vi "Autonomous Independent.vi"   [LabVIEW 2017]
doc: "This VI is called when autonomous begins, and will automatically be terminated when autonomous ends. You can carry out timed or sensor driven robot movement independently without needing to return to the caller."
uses:
  <vilib>/Rock Robotics/WPI/SafetyOutput/WPI_SafetyOutputConfigMenu.ctl
  <vilib>/Rock Robotics/WPI/ThirdParty/Phoenix-LabVIEW/Motor Controller/Controls/CTRE_Phoenix_MotorControl_ControlMode.ctl
  <vilib>/Rock Robotics/WPI/Utilities/WPI_GetSetVariantRefNum.vi
  Robot Global Data.vi
  <vilib>/Rock Robotics/WPI/RobotDrive/WPI_RobotDriveArcadeDrive_Standard(NoSaturation).vi
  <vilib>/Rock Robotics/WPI/RobotDrive/WPI_RobotDriveMecanumDrive_Cartesian.vi
  <vilib>/Rock Robotics/WPI/RobotDrive/WPI_RobotDriveMecanumDrive_Polar.vi
panel:
  # "Be sure to right-click and choose Data Operations>>Make Current Value default if you want to save the array values with the VI"
types:
  T1 = typedef "WPI_SafetyOutputConfigMenu.ctl" = enum16{"Enable", "Disable"}
  T2 = typedef "WPI_RobotDriveDevRef.ctl" = cluster{"DevStatus":errorcluster, "Motors[]":T3[], "Square Inputs":bool, "Max Output":dbl}
  T3 = typedef "WPI_MotorControlDeviceRef.ctl" = cluster{"DeviceStatus":errorcluster, "Type":T4, "PWM":cluster{"PWM Channel":T5, "DeadBand":T6}, "CAN":cluster{"Device Number":u8, "SetOutput VI Ref":variant, "GetOutput VI Ref":variant, "Enable VI Ref":variant, "Disable VI Ref":variant, "Data":variant}, "Invert":bool, "DIO PWM":cluster{"PWM \"Enable\" Channel":T5, "DIOChannel":T7, "PWM Rate":dbl}}
  T4 = typedef "WPI_MotorControlType.ctl" = enum16{"PWM", "CAN", "DIO PWM"}
  T5 = typedef "FPGA_DIOPWMChannel.ctl" = enum8{"PWM 0", "PWM 1", "PWM 2", "PWM 3", "PWM 4", "PWM 5", "PWM 6", "PWM 7", "PWM 8", "PWM 9", "PWM MXP 0", "PWM MXP 1", "PWM MXP 2", "PWM MXP 3", "PWM MXP 4", "PWM MXP 5", "PWM MXP 6", "PWM MXP 7", "PWM MXP 8", "PWM MXP 9", "Invalid"}
  T6 = typedef "WPI_PWMDeadband.ctl" = cluster{"Name":string, "maxPositivePwm":i32, "minPositivePwm":i32, "centerPwm":i32, "maxNegativePwm":i32, "minNegativePwm":i32, "angularRange":u16}
  T7 = typedef "FPGA_DIOChannel.ctl" = enum8{"DIO 0", "DIO 1", "DIO 2", "DIO 3", "DIO 4", "DIO 5", "DIO 6", "DIO 7", "DIO 8", "DIO 9", "DIO MXP 0", "DIO MXP 1", "DIO MXP 2", "DIO MXP 3", "DIO MXP 4", "DIO MXP 5", "DIO MXP 6", "DIO MXP 7", "DIO MXP 8", "DIO MXP 9", "DIO MXP 10", "DIO MXP 11", "DIO MXP 12", "DIO MXP 13", "DIO MXP 14", "DIO MXP 15", "SPI Port CS1", "SPI Port CS2", "SPI Port CS3", "SPI Port MISO", "SPI Port MOSI", "Invalid"}
  T8 = typedef "CTRE_Phoenix_MotorControl_ControlMode.ctl" = u16
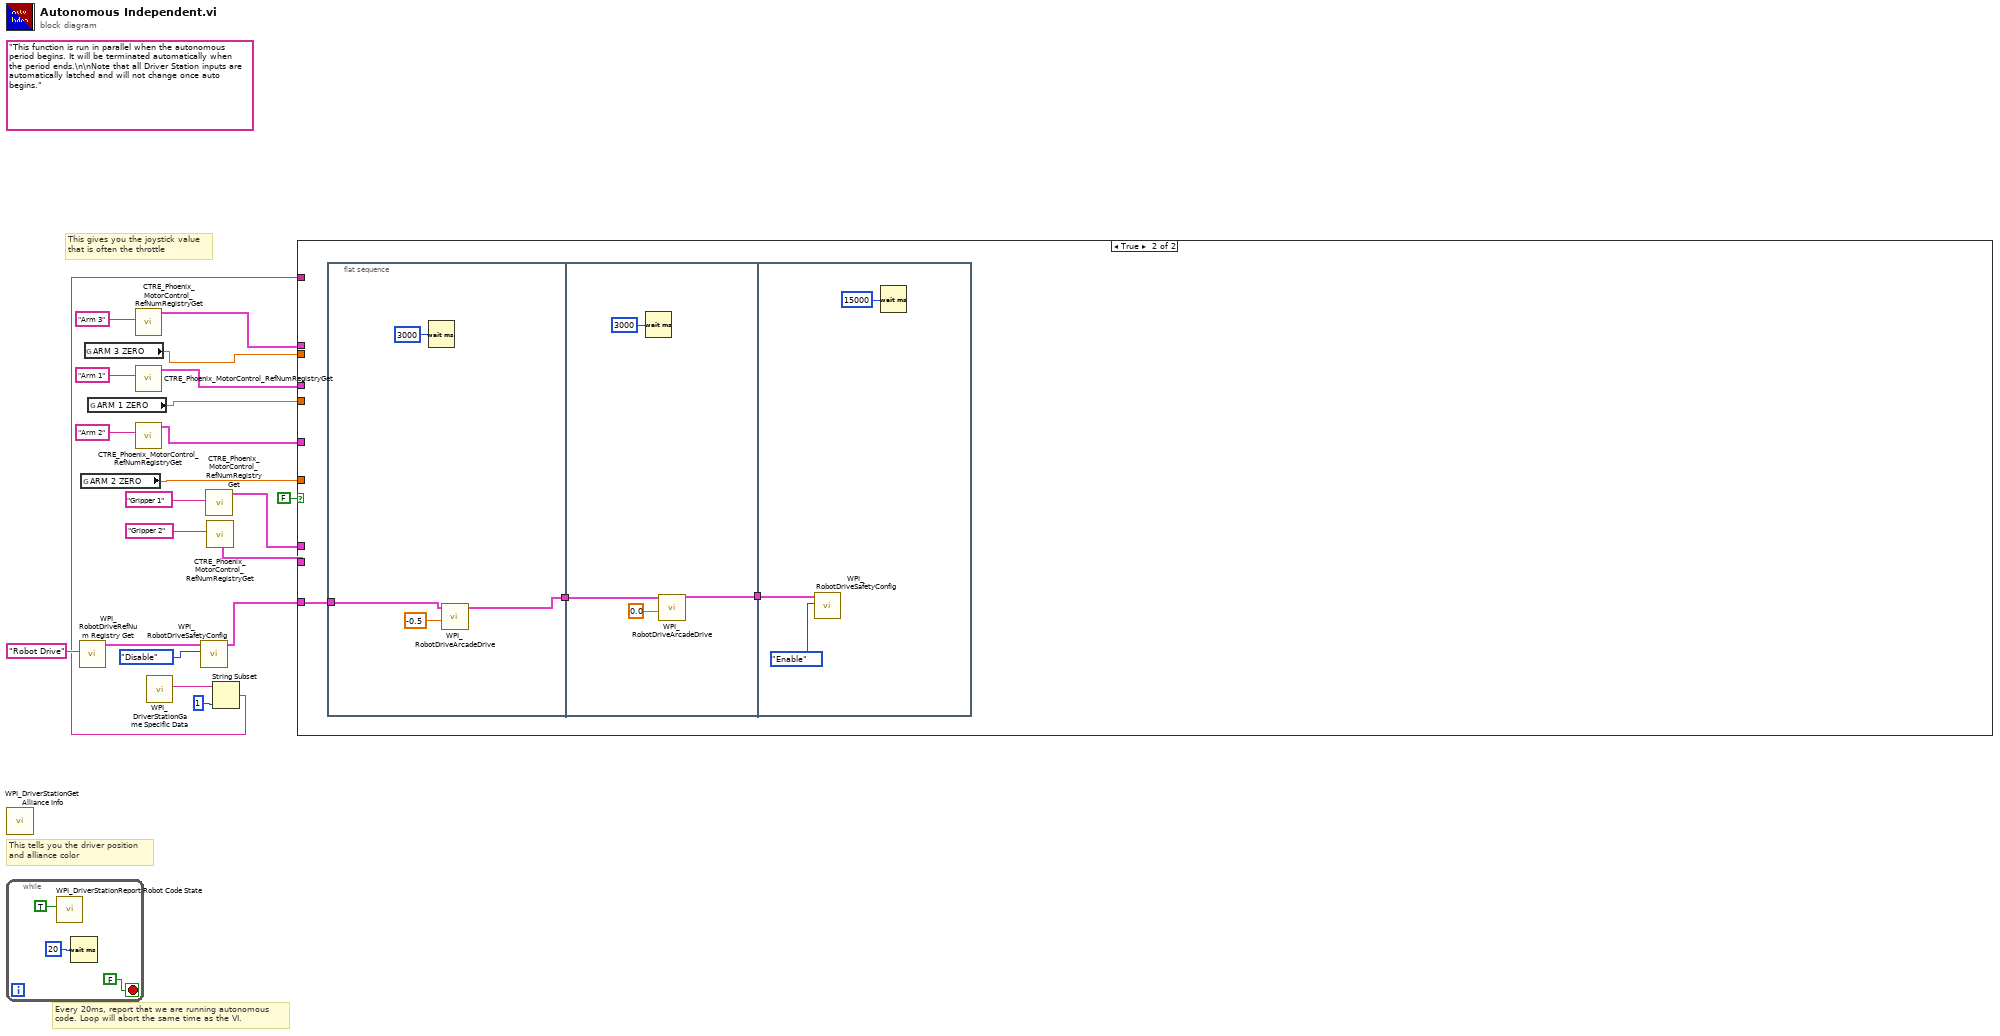
[diagram p0: block diagram]
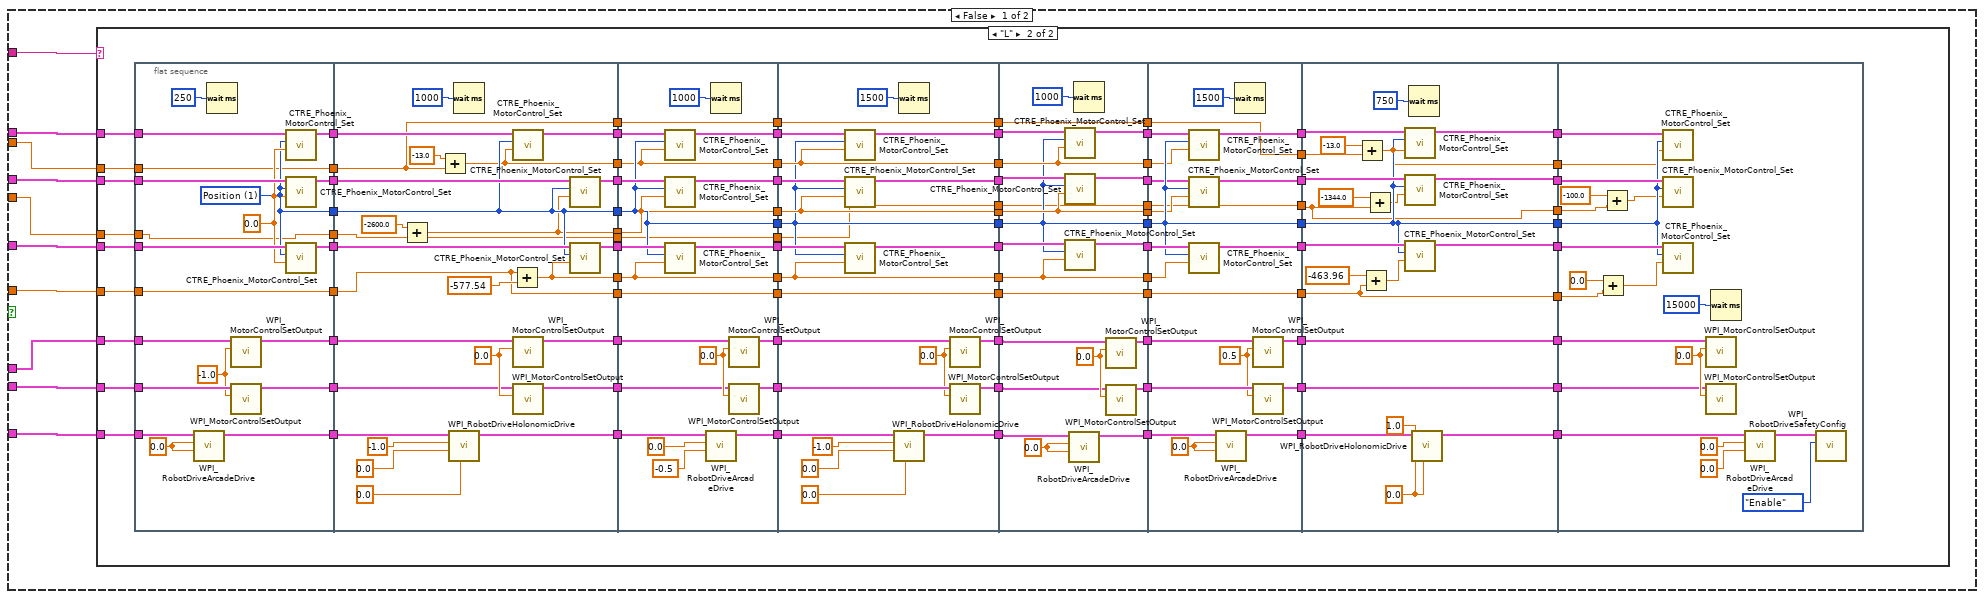
[diagram p2: hidden frame]
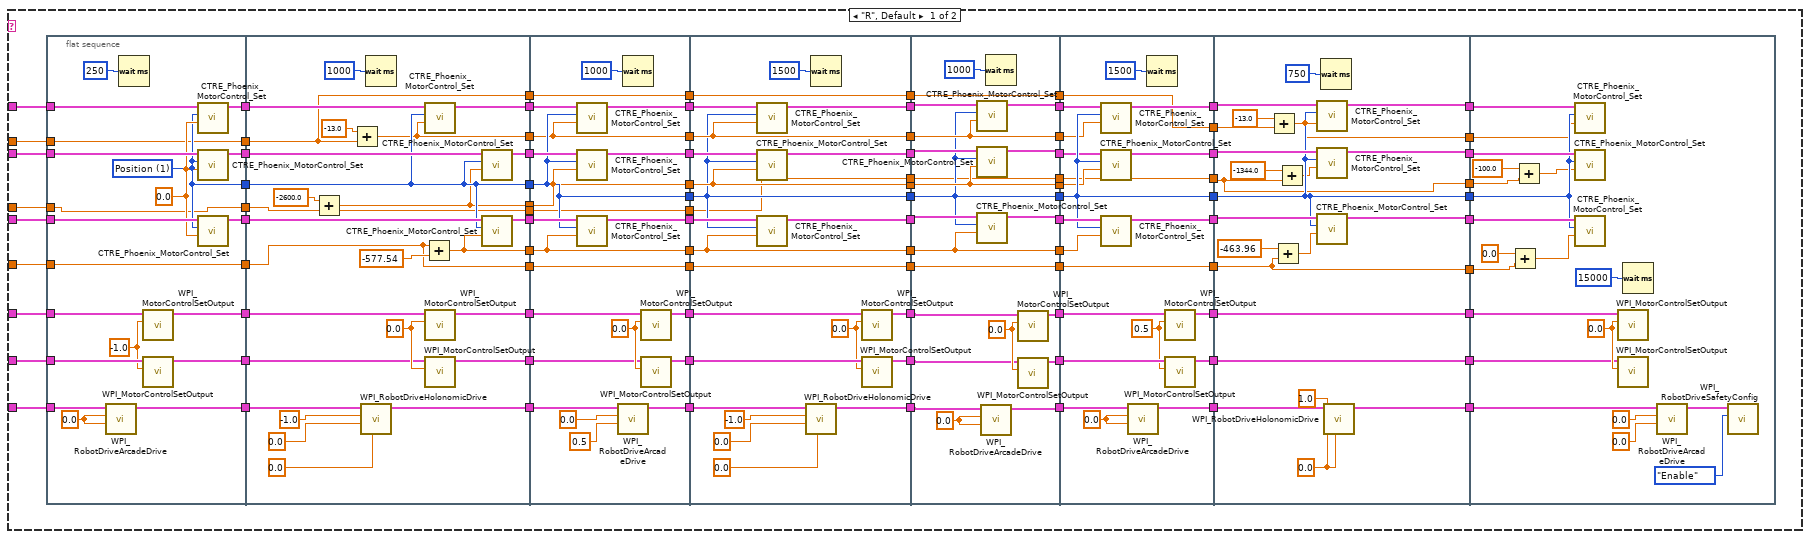
[diagram p3: hidden frame]
diagram:
  (unwired) "This function is run in parallel when the autonomous period begins. It will be terminated automatically when the period ends.\n\nNote that all Driver Station inputs are automatically latched and will not change once auto begins."
  # "Every 20ms, report that we are running autonomous\ncode. Loop will abort the same time as the VI."
  # "This gives you the joystick value\nthat is often the throttle"
  # "This tells you the driver position\nand alliance color"
  n1 = call <vilib>:"WPI_DriverStationGet Alliance Info.vi"() -> ()  [unwired: 12 out]
  n2 = while {
    stop <- FALSE stop-if-true
    n3 = call <vilib>:"WPI_DriverStationReport Robot Code State.vi"("Autonomous"=TRUE) -> ()  [unwired: 10 in, 1 out]
    n4 = Wait (ms)(milliseconds to wait=u32 20) -> ()  [unwired: 1 out]
  }
  n5 = call <vilib>:"WPI_RobotDriveRefNum Registry Get.vi"("refnum name"="Robot Drive") -> ("RobotDriveDevRef"=w17:T2)  [unwired: 1 in, 9 out]
  n6 = global read "Robot Global Data.vi" "ARM 2 ZERO"() -> (w4:dbl)
  n7 = global read "Robot Global Data.vi" "ARM 3 ZERO"() -> (w2:dbl)
  n8 = global read "Robot Global Data.vi" "ARM 1 ZERO"() -> (w3:dbl)
  n9 = call <vilib>:"CTRE_Phoenix_MotorControl_RefNumRegistryGet.vi"("refnum name"="Arm 3") -> ("PhoenixMotorControlDevRef"=w5:T3)  [unwired: 9 in, 1 out]
  n10 = call <vilib>:"CTRE_Phoenix_MotorControl_RefNumRegistryGet.vi"("refnum name"="Arm 1") -> ("PhoenixMotorControlDevRef"=w7:T3)  [unwired: 9 in, 1 out]
  n11 = call <vilib>:"CTRE_Phoenix_MotorControl_RefNumRegistryGet.vi"("refnum name"="Arm 2") -> ("PhoenixMotorControlDevRef"=w6:T3)  [unwired: 9 in, 1 out]
  n12 = call <vilib>:"WPI_DriverStationGame Specific Data.vi"() -> ("Game Specific Data"=w20:string)  [unwired: 11 in]
  n13 = call <vilib>:"WPI_RobotDriveSafetyConfig.vi"("mode"=WPI_SafetyOutputConfigMenu."Disable", "RobotDriveDevRef"=w17) -> ("RobotDriveDevRef"=w15:T2)  [unwired: 8 in, 1 out]
  n14 = call <vilib>:"CTRE_Phoenix_MotorControl_RefNumRegistryGet.vi"("refnum name"="Gripper 1") -> ("PhoenixMotorControlDevRef"=w12:T3)  [unwired: 9 in, 1 out]
  n15 = call <vilib>:"CTRE_Phoenix_MotorControl_RefNumRegistryGet.vi"("refnum name"="Gripper 2") -> ("PhoenixMotorControlDevRef"=w11:T3)  [unwired: 9 in, 1 out]
  n16 = String Subset(string=w20, length (rest)=1 ("length (rest)")) -> (substring=w18:string)  [unwired: 1 in]
  n17 = case shown="True" FALSE {
    tunnel: w18 -> [w34 _]
    tunnel: w15 -> [w33 w581]
    tunnel: w12 -> [w32 _]
    tunnel: w11 -> [w31 _]
    tunnel: w7 -> [w30 _]
    tunnel: w6 -> [w29 _]
    tunnel: w5 -> [w28 _]
    tunnel: w4 -> [w27 _]
    tunnel: w3 -> [w26 _]
    tunnel: w2 -> [w25 _]
    frame False {
      n18 = case shown="\"L\"" w34 {
        tunnel: w33 -> [w125 w397]
        tunnel: w32 -> [w124 w396]
        tunnel: w31 -> [w123 w395]
        tunnel: w28 -> [w120 w392]
        tunnel: w30 -> [w119 w391]
        tunnel: w29 -> [w118 w390]
        tunnel: w27 -> [w113 w385]
        tunnel: w26 -> [w110 w382]
        tunnel: w25 -> [w100 w372]
        frame "R", Default {
          n19 = flat-sequence {
            tunnel: w125 -> [w144]
            tunnel: w124 -> [w142]
            tunnel: w123 -> [w141]
            tunnel: [w139] -> w122
            tunnel: [w138] -> w121
            tunnel: w120 -> [w137]
            tunnel: w119 -> [w136]
            tunnel: w118 -> [w135]
            tunnel: [w133] -> w117
            tunnel: [w132] -> w116
            tunnel: [w131] -> w115
            tunnel: [w130] -> w114
            tunnel: w113 -> [w129]
            tunnel: [w129] -> w112
            tunnel: [w128] -> w111
            tunnel: w110 -> [w128]
            tunnel: [w127] -> w109
            tunnel: [w126] -> w101
            tunnel: w100 -> [w126]
            tunnel: [w160] -> w108
            tunnel: [w159] -> w107
            tunnel: [w158] -> w106
            tunnel: [w157] -> w105
            tunnel: [w156] -> w104
            tunnel: [w155] -> w103
            tunnel: [w154] -> w102
            tunnel: [w152] -> w99
            tunnel: [w151] -> w98
            tunnel: [w150] -> w97
            tunnel: w101 -> [w146]
            tunnel: w109 -> [w163]
            tunnel: w111 -> [w147]
            tunnel: w112 -> [w148]
            tunnel: w114 -> [w170]
            tunnel: w115 -> [w156]
            tunnel: w116 -> [w172]
            tunnel: w117 -> [w171]
            tunnel: w121 -> [w165]
            tunnel: w122 -> [w164]
            tunnel: [w148] -> w48
            tunnel: [w147] -> w43
            tunnel: [w146] -> w38
            tunnel: w108 -> [w195]
            tunnel: w107 -> [w192]
            tunnel: w106 -> [w191]
            tunnel: w105 -> [w190]
            tunnel: w104 -> [w182]
            tunnel: w103 -> [w188]
            tunnel: w102 -> [w187]
            tunnel: [w186] -> w96
            tunnel: [w185] -> w95
            tunnel: [w184] -> w94
            tunnel: [w183] -> w93
            tunnel: [w182] -> w92
            tunnel: [w181] -> w91
            tunnel: [w180] -> w90
            tunnel: w99 -> [w176]
            tunnel: w98 -> [w177]
            tunnel: w97 -> [w178]
            tunnel: [w178] -> w89
            tunnel: [w177] -> w88
            tunnel: [w176] -> w87
            tunnel: [w175] -> w49
            tunnel: w48 -> [w175]
            tunnel: [w174] -> w44
            tunnel: w43 -> [w174]
            tunnel: [w173] -> w39
            tunnel: w38 -> [w173]
            tunnel: w96 -> [w213]
            tunnel: w95 -> [w212]
            tunnel: [w211] -> w86
            tunnel: w94 -> [w214]
            tunnel: [w209] -> w84
            tunnel: w93 -> [w199]
            tunnel: w92 -> [w205]
            tunnel: [w205] -> w82
            tunnel: w91 -> [w219]
            tunnel: [w216] -> w80
            tunnel: w90 -> [w218]
            tunnel: [w217] -> w78
            tunnel: w89 -> [w206]
            tunnel: [w206] -> w76
            tunnel: w88 -> [w207]
            tunnel: [w207] -> w74
            tunnel: w87 -> [w208]
            tunnel: [w208] -> w72
            tunnel: [w210] -> w70
            tunnel: [w200] -> w68
            tunnel: [w198] -> w50
            tunnel: w49 -> [w198]
            tunnel: [w197] -> w45
            tunnel: w44 -> [w197]
            tunnel: [w196] -> w40
            tunnel: w39 -> [w196]
            tunnel: w86 -> [w240]
            tunnel: [w241] -> w85
            tunnel: w84 -> [w238]
            tunnel: [w237] -> w83
            tunnel: w82 -> [w233]
            tunnel: [w233] -> w81
            tunnel: w80 -> [w227]
            tunnel: [w225] -> w79
            tunnel: w78 -> [w226]
            tunnel: [w229] -> w77
            tunnel: w76 -> [w232]
            tunnel: [w232] -> w75
            tunnel: w74 -> [w235]
            tunnel: [w235] -> w73
            tunnel: w72 -> [w234]
            tunnel: [w234] -> w71
            tunnel: w70 -> [w239]
            tunnel: [w236] -> w69
            tunnel: w68 -> [w228]
            tunnel: [w224] -> w67
            tunnel: [w222] -> w51
            tunnel: w50 -> [w222]
            tunnel: [w221] -> w46
            tunnel: w45 -> [w221]
            tunnel: [w220] -> w41
            tunnel: w40 -> [w220]
            tunnel: [w256] -> w66
            tunnel: w85 -> [w254]
            tunnel: [w255] -> w64
            tunnel: w83 -> [w258]
            tunnel: [w257] -> w62
            tunnel: [w247] -> w60
            tunnel: w81 -> [w253]
            tunnel: [w253] -> w58
            tunnel: w79 -> [w261]
            tunnel: [w260] -> w56
            tunnel: w77 -> [w263]
            tunnel: [w262] -> w54
            tunnel: w75 -> [w249]
            tunnel: w73 -> [w250]
            tunnel: w71 -> [w251]
            tunnel: w69 -> [w252]
            tunnel: w67 -> [w246]
            tunnel: [w244] -> w52
            tunnel: w51 -> [w244]
            tunnel: [w243] -> w47
            tunnel: w46 -> [w243]
            tunnel: [w242] -> w42
            tunnel: w41 -> [w242]
            tunnel: w66 -> [w277]
            tunnel: [w276] -> w65
            tunnel: w64 -> [w275]
            tunnel: [w274] -> w63
            tunnel: w62 -> [w279]
            tunnel: [w278] -> w61
            tunnel: w60 -> [w286]
            tunnel: [w283] -> w59
            tunnel: w58 -> [w273]
            tunnel: [w273] -> w57
            tunnel: w56 -> [w285]
            tunnel: [w285] -> w55
            tunnel: w54 -> [w284]
            tunnel: [w284] -> w53
            tunnel: w52 -> [w268]
            tunnel: w47 -> [w267]
            tunnel: w42 -> [w265]
            tunnel: [w268] -> w37
            tunnel: [w267] -> w36
            tunnel: [w264] -> w35
            tunnel: w65 -> [w303]
            tunnel: w63 -> [w302]
            tunnel: w61 -> [w301]
            tunnel: w59 -> [w300]
            tunnel: w57 -> [w297]
            tunnel: w55 -> [w299]
            tunnel: w53 -> [w298]
            tunnel: w37 -> [w292]
            tunnel: w36 -> [w289]
            tunnel: w35 -> [w288]
            frame #0 {
              w131 = T8 1 items=["PercentOutput"=0, "Position"=1, "Velocity"=2, "Current"=3, "Follower"=5, "MotionProfile"=6, "MotionMagic"=7, "MotionMagicArc"=8, "MotionProfileArc"=10, "Disabled"=15] ("Control Mode")
              w134 = 0.0 ("Output")
              w140 = -1.0 ("Output")
              w143 = 0.0 ("X axis value")
              n20 = call-poly <vilib>:"WPI_RobotDriveArcadeDrive.vi"("Y axis value"=w143, "X axis value"=w143, "RobotDriveDevRef"=w144) -> ("RobotDriveDevRef"=w127:T2)  [unwired: 6 in, 2 out]
              n21 = Wait (ms)(milliseconds to wait=u32 250) -> ()  [unwired: 1 out]
              n22 = call <vilib>:"WPI_MotorControlSetOutput.vi"("Output"=w140, "MotorControlDevRef"=w142) -> ("MotorControlDevRef"=w139:T3)  [unwired: 7 in, 2 out]
              n23 = call <vilib>:"WPI_MotorControlSetOutput.vi"("Output"=w140, "MotorControlDevRef"=w141) -> ("MotorControlDevRef"=w138:T3)  [unwired: 7 in, 2 out]
              n24 = call <vilib>:"CTRE_Phoenix_MotorControl_Set.vi"("Output"=w134, "Control Mode"=w131, "PhoenixMotorControlDevRef"=w137) -> ("PhoenixMotorControlDevRef"=w130:T3)  [unwired: 7 in, 1 out]
              n25 = call <vilib>:"CTRE_Phoenix_MotorControl_Set.vi"("Output"=w134, "Control Mode"=w131, "PhoenixMotorControlDevRef"=w136) -> ("PhoenixMotorControlDevRef"=w132:T3)  [unwired: 7 in, 1 out]
              n26 = call <vilib>:"CTRE_Phoenix_MotorControl_Set.vi"("Output"=w134, "Control Mode"=w131, "PhoenixMotorControlDevRef"=w135) -> ("PhoenixMotorControlDevRef"=w133:T3)  [unwired: 7 in, 1 out]
            }
            frame #1 {
              w166 = 0.0 ("Output")
              n27 = Add(x=-2600.0, y=w147) -> (x+y=w151:dbl)
              n28 = Add(x=-13.0 ("Output"), y=w146) -> (x+y=w152:dbl)
              n29 = call-poly <vilib>:"WPI_RobotDriveHolonomicDrive.vi"("Rotation"=0.0 ("Gyro Angle"), "Y"=0.0, "X"=-1.0, "RobotDriveDevRef"=w163) -> ("RobotDriveDevRef"=w160:T2)  [unwired: 5 in, 2 out]
              n30 = Wait (ms)(milliseconds to wait=u32 1000) -> ()  [unwired: 1 out]
              n31 = Add(x=w148, y=-577.54) -> (x+y=w150:dbl)
              n32 = call <vilib>:"CTRE_Phoenix_MotorControl_Set.vi"("Output"=w152, "Control Mode"=w156, "PhoenixMotorControlDevRef"=w170) -> ("PhoenixMotorControlDevRef"=w159:T3)  [unwired: 7 in, 1 out]
              n33 = call <vilib>:"WPI_MotorControlSetOutput.vi"("Output"=w166, "MotorControlDevRef"=w164) -> ("MotorControlDevRef"=w154:T3)  [unwired: 7 in, 2 out]
              n34 = call <vilib>:"WPI_MotorControlSetOutput.vi"("Output"=w166, "MotorControlDevRef"=w165) -> ("MotorControlDevRef"=w155:T3)  [unwired: 7 in, 2 out]
              n35 = call <vilib>:"CTRE_Phoenix_MotorControl_Set.vi"("Output"=w151, "Control Mode"=w156, "PhoenixMotorControlDevRef"=w172) -> ("PhoenixMotorControlDevRef"=w157:T3)  [unwired: 7 in, 1 out]
              n36 = call <vilib>:"CTRE_Phoenix_MotorControl_Set.vi"("Output"=w150, "Control Mode"=w156, "PhoenixMotorControlDevRef"=w171) -> ("PhoenixMotorControlDevRef"=w158:T3)  [unwired: 7 in, 1 out]
            }
            frame #2 {
              w189 = 0.0 ("Output")
              n37 = call <vilib>:"CTRE_Phoenix_MotorControl_Set.vi"("Output"=w176, "Control Mode"=w182, "PhoenixMotorControlDevRef"=w192) -> ("PhoenixMotorControlDevRef"=w184:T3)  [unwired: 7 in, 1 out]
              n38 = call <vilib>:"CTRE_Phoenix_MotorControl_Set.vi"("Output"=w177, "Control Mode"=w182, "PhoenixMotorControlDevRef"=w190) -> ("PhoenixMotorControlDevRef"=w186:T3)  [unwired: 7 in, 1 out]
              n39 = call <vilib>:"CTRE_Phoenix_MotorControl_Set.vi"("Output"=w178, "Control Mode"=w182, "PhoenixMotorControlDevRef"=w191) -> ("PhoenixMotorControlDevRef"=w185:T3)  [unwired: 7 in, 1 out]
              n40 = call-poly <vilib>:"WPI_RobotDriveArcadeDrive.vi"("Y axis value"=0.5, "X axis value"=0.0, "RobotDriveDevRef"=w195) -> ("RobotDriveDevRef"=w183:T2)  [unwired: 6 in, 2 out]
              n41 = Wait (ms)(milliseconds to wait=u32 1000) -> ()  [unwired: 1 out]
              n42 = call <vilib>:"WPI_MotorControlSetOutput.vi"("Output"=w189, "MotorControlDevRef"=w187) -> ("MotorControlDevRef"=w180:T3)  [unwired: 7 in, 2 out]
              n43 = call <vilib>:"WPI_MotorControlSetOutput.vi"("Output"=w189, "MotorControlDevRef"=w188) -> ("MotorControlDevRef"=w181:T3)  [unwired: 7 in, 2 out]
            }
            frame #3 {
              w215 = 0.0 ("Output")
              n44 = call <vilib>:"CTRE_Phoenix_MotorControl_Set.vi"("Output"=w208, "Control Mode"=w205, "PhoenixMotorControlDevRef"=w214) -> ("PhoenixMotorControlDevRef"=w209:T3)  [unwired: 7 in, 1 out]
              n45 = call <vilib>:"CTRE_Phoenix_MotorControl_Set.vi"("Output"=w207, "Control Mode"=w205, "PhoenixMotorControlDevRef"=w213) -> ("PhoenixMotorControlDevRef"=w210:T3)  [unwired: 7 in, 1 out]
              n46 = call <vilib>:"CTRE_Phoenix_MotorControl_Set.vi"("Output"=w206, "Control Mode"=w205, "PhoenixMotorControlDevRef"=w212) -> ("PhoenixMotorControlDevRef"=w211:T3)  [unwired: 7 in, 1 out]
              n47 = call-poly <vilib>:"WPI_RobotDriveHolonomicDrive.vi"("Rotation"=0.0 ("Gyro Angle"), "Y"=0.0, "X"=-1.0, "RobotDriveDevRef"=w199) -> ("RobotDriveDevRef"=w200:T2)  [unwired: 5 in, 2 out]
              n48 = Wait (ms)(milliseconds to wait=u32 1500) -> ()  [unwired: 1 out]
              n49 = call <vilib>:"WPI_MotorControlSetOutput.vi"("Output"=w215, "MotorControlDevRef"=w218) -> ("MotorControlDevRef"=w217:T3)  [unwired: 7 in, 2 out]
              n50 = call <vilib>:"WPI_MotorControlSetOutput.vi"("Output"=w215, "MotorControlDevRef"=w219) -> ("MotorControlDevRef"=w216:T3)  [unwired: 7 in, 2 out]
            }
            frame #4 {
              w231 = 0.0 ("X axis value")
              w230 = 0.0 ("Output")
              n51 = call <vilib>:"CTRE_Phoenix_MotorControl_Set.vi"("Output"=w234, "Control Mode"=w233, "PhoenixMotorControlDevRef"=w238) -> ("PhoenixMotorControlDevRef"=w237:T3)  [unwired: 7 in, 1 out]
              n52 = call <vilib>:"CTRE_Phoenix_MotorControl_Set.vi"("Output"=w235, "Control Mode"=w233, "PhoenixMotorControlDevRef"=w239) -> ("PhoenixMotorControlDevRef"=w236:T3)  [unwired: 7 in, 1 out]
              n53 = call <vilib>:"CTRE_Phoenix_MotorControl_Set.vi"("Output"=w232, "Control Mode"=w233, "PhoenixMotorControlDevRef"=w240) -> ("PhoenixMotorControlDevRef"=w241:T3)  [unwired: 7 in, 1 out]
              n54 = call-poly <vilib>:"WPI_RobotDriveArcadeDrive.vi"("Y axis value"=w231, "X axis value"=w231, "RobotDriveDevRef"=w228) -> ("RobotDriveDevRef"=w224:T2)  [unwired: 6 in, 2 out]
              n55 = Wait (ms)(milliseconds to wait=u32 1000) -> ()  [unwired: 1 out]
              n56 = call <vilib>:"WPI_MotorControlSetOutput.vi"("Output"=w230, "MotorControlDevRef"=w226) -> ("MotorControlDevRef"=w229:T3)  [unwired: 7 in, 2 out]
              n57 = call <vilib>:"WPI_MotorControlSetOutput.vi"("Output"=w230, "MotorControlDevRef"=w227) -> ("MotorControlDevRef"=w225:T3)  [unwired: 7 in, 2 out]
            }
            frame #5 {
              w245 = 0.0 ("X axis value")
              w259 = 0.5 ("Output")
              n58 = call <vilib>:"CTRE_Phoenix_MotorControl_Set.vi"("Output"=w251, "Control Mode"=w253, "PhoenixMotorControlDevRef"=w258) -> ("PhoenixMotorControlDevRef"=w257:T3)  [unwired: 7 in, 1 out]
              n59 = call <vilib>:"CTRE_Phoenix_MotorControl_Set.vi"("Output"=w250, "Control Mode"=w253, "PhoenixMotorControlDevRef"=w252) -> ("PhoenixMotorControlDevRef"=w256:T3)  [unwired: 7 in, 1 out]
              n60 = call <vilib>:"CTRE_Phoenix_MotorControl_Set.vi"("Output"=w249, "Control Mode"=w253, "PhoenixMotorControlDevRef"=w254) -> ("PhoenixMotorControlDevRef"=w255:T3)  [unwired: 7 in, 1 out]
              n61 = call-poly <vilib>:"WPI_RobotDriveArcadeDrive.vi"("Y axis value"=w245, "X axis value"=w245, "RobotDriveDevRef"=w246) -> ("RobotDriveDevRef"=w247:T2)  [unwired: 6 in, 2 out]
              n62 = Wait (ms)(milliseconds to wait=u32 1500) -> ()  [unwired: 1 out]
              n63 = call <vilib>:"WPI_MotorControlSetOutput.vi"("Output"=w259, "MotorControlDevRef"=w263) -> ("MotorControlDevRef"=w262:T3)  [unwired: 7 in, 2 out]
              n64 = call <vilib>:"WPI_MotorControlSetOutput.vi"("Output"=w259, "MotorControlDevRef"=w261) -> ("MotorControlDevRef"=w260:T3)  [unwired: 7 in, 2 out]
            }
            frame #6 {
              w281 = 0.0 ("Direction")
              n65 = Add(x=-13.0, y=w265) -> (x+y=w264:dbl)
              n66 = Add(x=-463.96, y=w268) -> (x+y=w272:dbl)
              n67 = Add(x=-1344.0, y=w267) -> (x+y=w269:dbl)
              n68 = call <vilib>:"CTRE_Phoenix_MotorControl_Set.vi"("Output"=w264, "Control Mode"=w273, "PhoenixMotorControlDevRef"=w279) -> ("PhoenixMotorControlDevRef"=w278:T3)  [unwired: 7 in, 1 out]
              n69 = call <vilib>:"CTRE_Phoenix_MotorControl_Set.vi"("Output"=w269, "Control Mode"=w273, "PhoenixMotorControlDevRef"=w277) -> ("PhoenixMotorControlDevRef"=w276:T3)  [unwired: 7 in, 1 out]
              n70 = call <vilib>:"CTRE_Phoenix_MotorControl_Set.vi"("Output"=w272, "Control Mode"=w273, "PhoenixMotorControlDevRef"=w275) -> ("PhoenixMotorControlDevRef"=w274:T3)  [unwired: 7 in, 1 out]
              n71 = Wait (ms)(milliseconds to wait=u32 750) -> ()  [unwired: 1 out]
              n72 = call-poly <vilib>:"WPI_RobotDriveHolonomicDrive.vi"("Rotation"=w281, "Direction"=w281, "Magnitude"=1.0, "RobotDriveDevRef"=w286) -> ("RobotDriveDevRef"=w283:T2)  [unwired: 5 in, 2 out]
            }
            frame #7 {
              w306 = 0.0 ("Output")
              n73 = Add(x=0.0, y=w292) -> (x+y=w293:dbl)
              n74 = Add(x=-100.0, y=w289) -> (x+y=w287:dbl)
              n75 = call <vilib>:"CTRE_Phoenix_MotorControl_Set.vi"("Output"=w288, "Control Mode"=w297, "PhoenixMotorControlDevRef"=w301) -> ()  [unwired: 7 in, 2 out]
              n76 = call <vilib>:"CTRE_Phoenix_MotorControl_Set.vi"("Output"=w287, "Control Mode"=w297, "PhoenixMotorControlDevRef"=w303) -> ()  [unwired: 7 in, 2 out]
              n77 = call <vilib>:"CTRE_Phoenix_MotorControl_Set.vi"("Output"=w293, "Control Mode"=w297, "PhoenixMotorControlDevRef"=w302) -> ()  [unwired: 7 in, 2 out]
              n78 = call <vilib>:"WPI_MotorControlSetOutput.vi"("Output"=w306, "MotorControlDevRef"=w298) -> ()  [unwired: 7 in, 3 out]
              n79 = call <vilib>:"WPI_MotorControlSetOutput.vi"("Output"=w306, "MotorControlDevRef"=w299) -> ()  [unwired: 7 in, 3 out]
              n80 = Wait (ms)(milliseconds to wait=u32 15000) -> ()  [unwired: 1 out]
              n81 = call-poly <vilib>:"WPI_RobotDriveArcadeDrive.vi"("Y axis value"=0.0, "X axis value"=0.0, "RobotDriveDevRef"=w300) -> ("RobotDriveDevRef"=w294:T2)  [unwired: 6 in, 2 out]
              n82 = call <vilib>:"WPI_RobotDriveSafetyConfig.vi"("mode"=WPI_SafetyOutputConfigMenu."Enable", "RobotDriveDevRef"=w294) -> ()  [unwired: 8 in, 2 out]
            }
          }
        }
        frame "L" {
          n83 = flat-sequence {
            tunnel: w397 -> [w416]
            tunnel: w396 -> [w414]
            tunnel: w395 -> [w413]
            tunnel: [w411] -> w394
            tunnel: [w410] -> w393
            tunnel: w392 -> [w409]
            tunnel: w391 -> [w408]
            tunnel: w390 -> [w407]
            tunnel: [w405] -> w389
            tunnel: [w404] -> w388
            tunnel: [w403] -> w387
            tunnel: [w402] -> w386
            tunnel: w385 -> [w401]
            tunnel: [w401] -> w384
            tunnel: [w400] -> w383
            tunnel: w382 -> [w400]
            tunnel: [w399] -> w381
            tunnel: [w398] -> w373
            tunnel: w372 -> [w398]
            tunnel: [w432] -> w380
            tunnel: [w431] -> w379
            tunnel: [w430] -> w378
            tunnel: [w429] -> w377
            tunnel: [w428] -> w376
            tunnel: [w427] -> w375
            tunnel: [w426] -> w374
            tunnel: [w424] -> w371
            tunnel: [w423] -> w370
            tunnel: [w422] -> w369
            tunnel: w373 -> [w418]
            tunnel: w381 -> [w435]
            tunnel: w383 -> [w419]
            tunnel: w384 -> [w420]
            tunnel: w386 -> [w442]
            tunnel: w387 -> [w428]
            tunnel: w388 -> [w444]
            tunnel: w389 -> [w443]
            tunnel: w393 -> [w437]
            tunnel: w394 -> [w436]
            tunnel: [w420] -> w320
            tunnel: [w419] -> w315
            tunnel: [w418] -> w310
            tunnel: w380 -> [w467]
            tunnel: w379 -> [w464]
            tunnel: w378 -> [w463]
            tunnel: w377 -> [w462]
            tunnel: w376 -> [w454]
            tunnel: w375 -> [w460]
            tunnel: w374 -> [w459]
            tunnel: [w458] -> w368
            tunnel: [w457] -> w367
            tunnel: [w456] -> w366
            tunnel: [w455] -> w365
            tunnel: [w454] -> w364
            tunnel: [w453] -> w363
            tunnel: [w452] -> w362
            tunnel: w371 -> [w448]
            tunnel: w370 -> [w449]
            tunnel: w369 -> [w450]
            tunnel: [w450] -> w361
            tunnel: [w449] -> w360
            tunnel: [w448] -> w359
            tunnel: [w447] -> w321
            tunnel: w320 -> [w447]
            tunnel: [w446] -> w316
            tunnel: w315 -> [w446]
            tunnel: [w445] -> w311
            tunnel: w310 -> [w445]
            tunnel: w368 -> [w485]
            tunnel: w367 -> [w484]
            tunnel: [w483] -> w358
            tunnel: w366 -> [w486]
            tunnel: [w481] -> w356
            tunnel: w365 -> [w471]
            tunnel: w364 -> [w477]
            tunnel: [w477] -> w354
            tunnel: w363 -> [w491]
            tunnel: [w488] -> w352
            tunnel: w362 -> [w490]
            tunnel: [w489] -> w350
            tunnel: w361 -> [w478]
            tunnel: [w478] -> w348
            tunnel: w360 -> [w479]
            tunnel: [w479] -> w346
            tunnel: w359 -> [w480]
            tunnel: [w480] -> w344
            tunnel: [w482] -> w342
            tunnel: [w472] -> w340
            tunnel: [w470] -> w322
            tunnel: w321 -> [w470]
            tunnel: [w469] -> w317
            tunnel: w316 -> [w469]
            tunnel: [w468] -> w312
            tunnel: w311 -> [w468]
            tunnel: w358 -> [w512]
            tunnel: [w513] -> w357
            tunnel: w356 -> [w510]
            tunnel: [w509] -> w355
            tunnel: w354 -> [w505]
            tunnel: [w505] -> w353
            tunnel: w352 -> [w499]
            tunnel: [w497] -> w351
            tunnel: w350 -> [w498]
            tunnel: [w501] -> w349
            tunnel: w348 -> [w504]
            tunnel: [w504] -> w347
            tunnel: w346 -> [w507]
            tunnel: [w507] -> w345
            tunnel: w344 -> [w506]
            tunnel: [w506] -> w343
            tunnel: w342 -> [w511]
            tunnel: [w508] -> w341
            tunnel: w340 -> [w500]
            tunnel: [w496] -> w339
            tunnel: [w494] -> w323
            tunnel: w322 -> [w494]
            tunnel: [w493] -> w318
            tunnel: w317 -> [w493]
            tunnel: [w492] -> w313
            tunnel: w312 -> [w492]
            tunnel: [w528] -> w338
            tunnel: w357 -> [w526]
            tunnel: [w527] -> w336
            tunnel: w355 -> [w530]
            tunnel: [w529] -> w334
            tunnel: [w519] -> w332
            tunnel: w353 -> [w525]
            tunnel: [w525] -> w330
            tunnel: w351 -> [w533]
            tunnel: [w532] -> w328
            tunnel: w349 -> [w535]
            tunnel: [w534] -> w326
            tunnel: w347 -> [w521]
            tunnel: w345 -> [w522]
            tunnel: w343 -> [w523]
            tunnel: w341 -> [w524]
            tunnel: w339 -> [w518]
            tunnel: [w516] -> w324
            tunnel: w323 -> [w516]
            tunnel: [w515] -> w319
            tunnel: w318 -> [w515]
            tunnel: [w514] -> w314
            tunnel: w313 -> [w514]
            tunnel: w338 -> [w549]
            tunnel: [w548] -> w337
            tunnel: w336 -> [w547]
            tunnel: [w546] -> w335
            tunnel: w334 -> [w551]
            tunnel: [w550] -> w333
            tunnel: w332 -> [w558]
            tunnel: [w555] -> w331
            tunnel: w330 -> [w545]
            tunnel: [w545] -> w329
            tunnel: w328 -> [w557]
            tunnel: [w557] -> w327
            tunnel: w326 -> [w556]
            tunnel: [w556] -> w325
            tunnel: w324 -> [w540]
            tunnel: w319 -> [w539]
            tunnel: w314 -> [w537]
            tunnel: [w540] -> w309
            tunnel: [w539] -> w308
            tunnel: [w536] -> w307
            tunnel: w337 -> [w575]
            tunnel: w335 -> [w574]
            tunnel: w333 -> [w573]
            tunnel: w331 -> [w572]
            tunnel: w329 -> [w569]
            tunnel: w327 -> [w571]
            tunnel: w325 -> [w570]
            tunnel: w309 -> [w564]
            tunnel: w308 -> [w561]
            tunnel: w307 -> [w560]
            frame #0 {
              w403 = T8 1 items=["PercentOutput"=0, "Position"=1, "Velocity"=2, "Current"=3, "Follower"=5, "MotionProfile"=6, "MotionMagic"=7, "MotionMagicArc"=8, "MotionProfileArc"=10, "Disabled"=15] ("Control Mode")
              w406 = 0.0 ("Output")
              w412 = -1.0 ("Output")
              w415 = 0.0 ("X axis value")
              n84 = call-poly <vilib>:"WPI_RobotDriveArcadeDrive.vi"("Y axis value"=w415, "X axis value"=w415, "RobotDriveDevRef"=w416) -> ("RobotDriveDevRef"=w399:T2)  [unwired: 6 in, 2 out]
              n85 = Wait (ms)(milliseconds to wait=u32 250) -> ()  [unwired: 1 out]
              n86 = call <vilib>:"WPI_MotorControlSetOutput.vi"("Output"=w412, "MotorControlDevRef"=w414) -> ("MotorControlDevRef"=w411:T3)  [unwired: 7 in, 2 out]
              n87 = call <vilib>:"WPI_MotorControlSetOutput.vi"("Output"=w412, "MotorControlDevRef"=w413) -> ("MotorControlDevRef"=w410:T3)  [unwired: 7 in, 2 out]
              n88 = call <vilib>:"CTRE_Phoenix_MotorControl_Set.vi"("Output"=w406, "Control Mode"=w403, "PhoenixMotorControlDevRef"=w409) -> ("PhoenixMotorControlDevRef"=w402:T3)  [unwired: 7 in, 1 out]
              n89 = call <vilib>:"CTRE_Phoenix_MotorControl_Set.vi"("Output"=w406, "Control Mode"=w403, "PhoenixMotorControlDevRef"=w408) -> ("PhoenixMotorControlDevRef"=w404:T3)  [unwired: 7 in, 1 out]
              n90 = call <vilib>:"CTRE_Phoenix_MotorControl_Set.vi"("Output"=w406, "Control Mode"=w403, "PhoenixMotorControlDevRef"=w407) -> ("PhoenixMotorControlDevRef"=w405:T3)  [unwired: 7 in, 1 out]
            }
            frame #1 {
              w438 = 0.0 ("Output")
              n91 = Add(x=-2600.0, y=w419) -> (x+y=w423:dbl)
              n92 = Add(x=-13.0 ("Output"), y=w418) -> (x+y=w424:dbl)
              n93 = call-poly <vilib>:"WPI_RobotDriveHolonomicDrive.vi"("Rotation"=0.0 ("Gyro Angle"), "Y"=0.0, "X"=-1.0, "RobotDriveDevRef"=w435) -> ("RobotDriveDevRef"=w432:T2)  [unwired: 5 in, 2 out]
              n94 = Wait (ms)(milliseconds to wait=u32 1000) -> ()  [unwired: 1 out]
              n95 = Add(x=w420, y=-577.54) -> (x+y=w422:dbl)
              n96 = call <vilib>:"CTRE_Phoenix_MotorControl_Set.vi"("Output"=w424, "Control Mode"=w428, "PhoenixMotorControlDevRef"=w442) -> ("PhoenixMotorControlDevRef"=w431:T3)  [unwired: 7 in, 1 out]
              n97 = call <vilib>:"WPI_MotorControlSetOutput.vi"("Output"=w438, "MotorControlDevRef"=w436) -> ("MotorControlDevRef"=w426:T3)  [unwired: 7 in, 2 out]
              n98 = call <vilib>:"WPI_MotorControlSetOutput.vi"("Output"=w438, "MotorControlDevRef"=w437) -> ("MotorControlDevRef"=w427:T3)  [unwired: 7 in, 2 out]
              n99 = call <vilib>:"CTRE_Phoenix_MotorControl_Set.vi"("Output"=w423, "Control Mode"=w428, "PhoenixMotorControlDevRef"=w444) -> ("PhoenixMotorControlDevRef"=w429:T3)  [unwired: 7 in, 1 out]
              n100 = call <vilib>:"CTRE_Phoenix_MotorControl_Set.vi"("Output"=w422, "Control Mode"=w428, "PhoenixMotorControlDevRef"=w443) -> ("PhoenixMotorControlDevRef"=w430:T3)  [unwired: 7 in, 1 out]
            }
            frame #2 {
              w461 = 0.0 ("Output")
              n101 = call <vilib>:"CTRE_Phoenix_MotorControl_Set.vi"("Output"=w448, "Control Mode"=w454, "PhoenixMotorControlDevRef"=w464) -> ("PhoenixMotorControlDevRef"=w456:T3)  [unwired: 7 in, 1 out]
              n102 = call <vilib>:"CTRE_Phoenix_MotorControl_Set.vi"("Output"=w449, "Control Mode"=w454, "PhoenixMotorControlDevRef"=w462) -> ("PhoenixMotorControlDevRef"=w458:T3)  [unwired: 7 in, 1 out]
              n103 = call <vilib>:"CTRE_Phoenix_MotorControl_Set.vi"("Output"=w450, "Control Mode"=w454, "PhoenixMotorControlDevRef"=w463) -> ("PhoenixMotorControlDevRef"=w457:T3)  [unwired: 7 in, 1 out]
              n104 = call-poly <vilib>:"WPI_RobotDriveArcadeDrive.vi"("Y axis value"=-0.5, "X axis value"=0.0, "RobotDriveDevRef"=w467) -> ("RobotDriveDevRef"=w455:T2)  [unwired: 6 in, 2 out]
              n105 = Wait (ms)(milliseconds to wait=u32 1000) -> ()  [unwired: 1 out]
              n106 = call <vilib>:"WPI_MotorControlSetOutput.vi"("Output"=w461, "MotorControlDevRef"=w459) -> ("MotorControlDevRef"=w452:T3)  [unwired: 7 in, 2 out]
              n107 = call <vilib>:"WPI_MotorControlSetOutput.vi"("Output"=w461, "MotorControlDevRef"=w460) -> ("MotorControlDevRef"=w453:T3)  [unwired: 7 in, 2 out]
            }
            frame #3 {
              w487 = 0.0 ("Output")
              n108 = call <vilib>:"CTRE_Phoenix_MotorControl_Set.vi"("Output"=w480, "Control Mode"=w477, "PhoenixMotorControlDevRef"=w486) -> ("PhoenixMotorControlDevRef"=w481:T3)  [unwired: 7 in, 1 out]
              n109 = call <vilib>:"CTRE_Phoenix_MotorControl_Set.vi"("Output"=w479, "Control Mode"=w477, "PhoenixMotorControlDevRef"=w485) -> ("PhoenixMotorControlDevRef"=w482:T3)  [unwired: 7 in, 1 out]
              n110 = call <vilib>:"CTRE_Phoenix_MotorControl_Set.vi"("Output"=w478, "Control Mode"=w477, "PhoenixMotorControlDevRef"=w484) -> ("PhoenixMotorControlDevRef"=w483:T3)  [unwired: 7 in, 1 out]
              n111 = call-poly <vilib>:"WPI_RobotDriveHolonomicDrive.vi"("Rotation"=0.0 ("Gyro Angle"), "Y"=0.0, "X"=-1.0, "RobotDriveDevRef"=w471) -> ("RobotDriveDevRef"=w472:T2)  [unwired: 5 in, 2 out]
              n112 = Wait (ms)(milliseconds to wait=u32 1500) -> ()  [unwired: 1 out]
              n113 = call <vilib>:"WPI_MotorControlSetOutput.vi"("Output"=w487, "MotorControlDevRef"=w490) -> ("MotorControlDevRef"=w489:T3)  [unwired: 7 in, 2 out]
              n114 = call <vilib>:"WPI_MotorControlSetOutput.vi"("Output"=w487, "MotorControlDevRef"=w491) -> ("MotorControlDevRef"=w488:T3)  [unwired: 7 in, 2 out]
            }
            frame #4 {
              w503 = 0.0 ("X axis value")
              w502 = 0.0 ("Output")
              n115 = call <vilib>:"CTRE_Phoenix_MotorControl_Set.vi"("Output"=w506, "Control Mode"=w505, "PhoenixMotorControlDevRef"=w510) -> ("PhoenixMotorControlDevRef"=w509:T3)  [unwired: 7 in, 1 out]
              n116 = call <vilib>:"CTRE_Phoenix_MotorControl_Set.vi"("Output"=w507, "Control Mode"=w505, "PhoenixMotorControlDevRef"=w511) -> ("PhoenixMotorControlDevRef"=w508:T3)  [unwired: 7 in, 1 out]
              n117 = call <vilib>:"CTRE_Phoenix_MotorControl_Set.vi"("Output"=w504, "Control Mode"=w505, "PhoenixMotorControlDevRef"=w512) -> ("PhoenixMotorControlDevRef"=w513:T3)  [unwired: 7 in, 1 out]
              n118 = call-poly <vilib>:"WPI_RobotDriveArcadeDrive.vi"("Y axis value"=w503, "X axis value"=w503, "RobotDriveDevRef"=w500) -> ("RobotDriveDevRef"=w496:T2)  [unwired: 6 in, 2 out]
              n119 = Wait (ms)(milliseconds to wait=u32 1000) -> ()  [unwired: 1 out]
              n120 = call <vilib>:"WPI_MotorControlSetOutput.vi"("Output"=w502, "MotorControlDevRef"=w498) -> ("MotorControlDevRef"=w501:T3)  [unwired: 7 in, 2 out]
              n121 = call <vilib>:"WPI_MotorControlSetOutput.vi"("Output"=w502, "MotorControlDevRef"=w499) -> ("MotorControlDevRef"=w497:T3)  [unwired: 7 in, 2 out]
            }
            frame #5 {
              w517 = 0.0 ("X axis value")
              w531 = 0.5 ("Output")
              n122 = call <vilib>:"CTRE_Phoenix_MotorControl_Set.vi"("Output"=w523, "Control Mode"=w525, "PhoenixMotorControlDevRef"=w530) -> ("PhoenixMotorControlDevRef"=w529:T3)  [unwired: 7 in, 1 out]
              n123 = call <vilib>:"CTRE_Phoenix_MotorControl_Set.vi"("Output"=w522, "Control Mode"=w525, "PhoenixMotorControlDevRef"=w524) -> ("PhoenixMotorControlDevRef"=w528:T3)  [unwired: 7 in, 1 out]
              n124 = call <vilib>:"CTRE_Phoenix_MotorControl_Set.vi"("Output"=w521, "Control Mode"=w525, "PhoenixMotorControlDevRef"=w526) -> ("PhoenixMotorControlDevRef"=w527:T3)  [unwired: 7 in, 1 out]
              n125 = call-poly <vilib>:"WPI_RobotDriveArcadeDrive.vi"("Y axis value"=w517, "X axis value"=w517, "RobotDriveDevRef"=w518) -> ("RobotDriveDevRef"=w519:T2)  [unwired: 6 in, 2 out]
              n126 = Wait (ms)(milliseconds to wait=u32 1500) -> ()  [unwired: 1 out]
              n127 = call <vilib>:"WPI_MotorControlSetOutput.vi"("Output"=w531, "MotorControlDevRef"=w535) -> ("MotorControlDevRef"=w534:T3)  [unwired: 7 in, 2 out]
              n128 = call <vilib>:"WPI_MotorControlSetOutput.vi"("Output"=w531, "MotorControlDevRef"=w533) -> ("MotorControlDevRef"=w532:T3)  [unwired: 7 in, 2 out]
            }
            frame #6 {
              w553 = 0.0 ("Direction")
              n129 = Add(x=-13.0, y=w537) -> (x+y=w536:dbl)
              n130 = Add(x=-463.96, y=w540) -> (x+y=w544:dbl)
              n131 = Add(x=-1344.0, y=w539) -> (x+y=w541:dbl)
              n132 = call <vilib>:"CTRE_Phoenix_MotorControl_Set.vi"("Output"=w536, "Control Mode"=w545, "PhoenixMotorControlDevRef"=w551) -> ("PhoenixMotorControlDevRef"=w550:T3)  [unwired: 7 in, 1 out]
              n133 = call <vilib>:"CTRE_Phoenix_MotorControl_Set.vi"("Output"=w541, "Control Mode"=w545, "PhoenixMotorControlDevRef"=w549) -> ("PhoenixMotorControlDevRef"=w548:T3)  [unwired: 7 in, 1 out]
              n134 = call <vilib>:"CTRE_Phoenix_MotorControl_Set.vi"("Output"=w544, "Control Mode"=w545, "PhoenixMotorControlDevRef"=w547) -> ("PhoenixMotorControlDevRef"=w546:T3)  [unwired: 7 in, 1 out]
              n135 = Wait (ms)(milliseconds to wait=u32 750) -> ()  [unwired: 1 out]
              n136 = call-poly <vilib>:"WPI_RobotDriveHolonomicDrive.vi"("Rotation"=w553, "Direction"=w553, "Magnitude"=1.0, "RobotDriveDevRef"=w558) -> ("RobotDriveDevRef"=w555:T2)  [unwired: 5 in, 2 out]
            }
            frame #7 {
              w578 = 0.0 ("Output")
              n137 = Add(x=0.0, y=w564) -> (x+y=w565:dbl)
              n138 = Add(x=-100.0, y=w561) -> (x+y=w559:dbl)
              n139 = call <vilib>:"CTRE_Phoenix_MotorControl_Set.vi"("Output"=w560, "Control Mode"=w569, "PhoenixMotorControlDevRef"=w573) -> ()  [unwired: 7 in, 2 out]
              n140 = call <vilib>:"CTRE_Phoenix_MotorControl_Set.vi"("Output"=w559, "Control Mode"=w569, "PhoenixMotorControlDevRef"=w575) -> ()  [unwired: 7 in, 2 out]
              n141 = call <vilib>:"CTRE_Phoenix_MotorControl_Set.vi"("Output"=w565, "Control Mode"=w569, "PhoenixMotorControlDevRef"=w574) -> ()  [unwired: 7 in, 2 out]
              n142 = call <vilib>:"WPI_MotorControlSetOutput.vi"("Output"=w578, "MotorControlDevRef"=w570) -> ()  [unwired: 7 in, 3 out]
              n143 = call <vilib>:"WPI_MotorControlSetOutput.vi"("Output"=w578, "MotorControlDevRef"=w571) -> ()  [unwired: 7 in, 3 out]
              n144 = Wait (ms)(milliseconds to wait=u32 15000) -> ()  [unwired: 1 out]
              n145 = call-poly <vilib>:"WPI_RobotDriveArcadeDrive.vi"("Y axis value"=0.0, "X axis value"=0.0, "RobotDriveDevRef"=w572) -> ("RobotDriveDevRef"=w566:T2)  [unwired: 6 in, 2 out]
              n146 = call <vilib>:"WPI_RobotDriveSafetyConfig.vi"("mode"=WPI_SafetyOutputConfigMenu."Enable", "RobotDriveDevRef"=w566) -> ()  [unwired: 8 in, 2 out]
            }
          }
        }
      }
    }
    frame True {
      n147 = flat-sequence {
        tunnel: w581 -> [w585]
        tunnel: [w582] -> w580
        tunnel: w580 -> [w587]
        tunnel: [w586] -> w579
        tunnel: w579 -> [w592]
        frame #0 {
          n148 = Wait (ms)(milliseconds to wait=u32 3000) -> ()  [unwired: 1 out]
          n149 = call-poly <vilib>:"WPI_RobotDriveArcadeDrive.vi"("Y axis value"=-0.5, "RobotDriveDevRef"=w585) -> ("RobotDriveDevRef"=w582:T2)  [unwired: 7 in, 2 out]
        }
        frame #1 {
          n150 = Wait (ms)(milliseconds to wait=u32 3000) -> ()  [unwired: 1 out]
          n151 = call-poly <vilib>:"WPI_RobotDriveArcadeDrive.vi"("Y axis value"=0.0, "RobotDriveDevRef"=w587) -> ("RobotDriveDevRef"=w586:T2)  [unwired: 7 in, 2 out]
        }
        frame #2 {
          n152 = call <vilib>:"WPI_RobotDriveSafetyConfig.vi"("mode"=WPI_SafetyOutputConfigMenu."Enable", "RobotDriveDevRef"=w592) -> ()  [unwired: 8 in, 2 out]
          n153 = Wait (ms)(milliseconds to wait=u32 15000) -> ()  [unwired: 1 out]
        }
      }
    }
  }
